vi "nipkg-updateControlFilePackageName.vi"(8 "error in (no error)":errorcluster, 9 "New Package Display Name":string, 10 "New Package Name":string, 11 "Package data":T1) -> (0 "error out":errorcluster, 3 "Package data out":T1)   [LabVIEW 2014, in "nipkg-build-system.lvlib"]
uses:
  nipkg-build-system.lvlib
  types/Package data.ctl
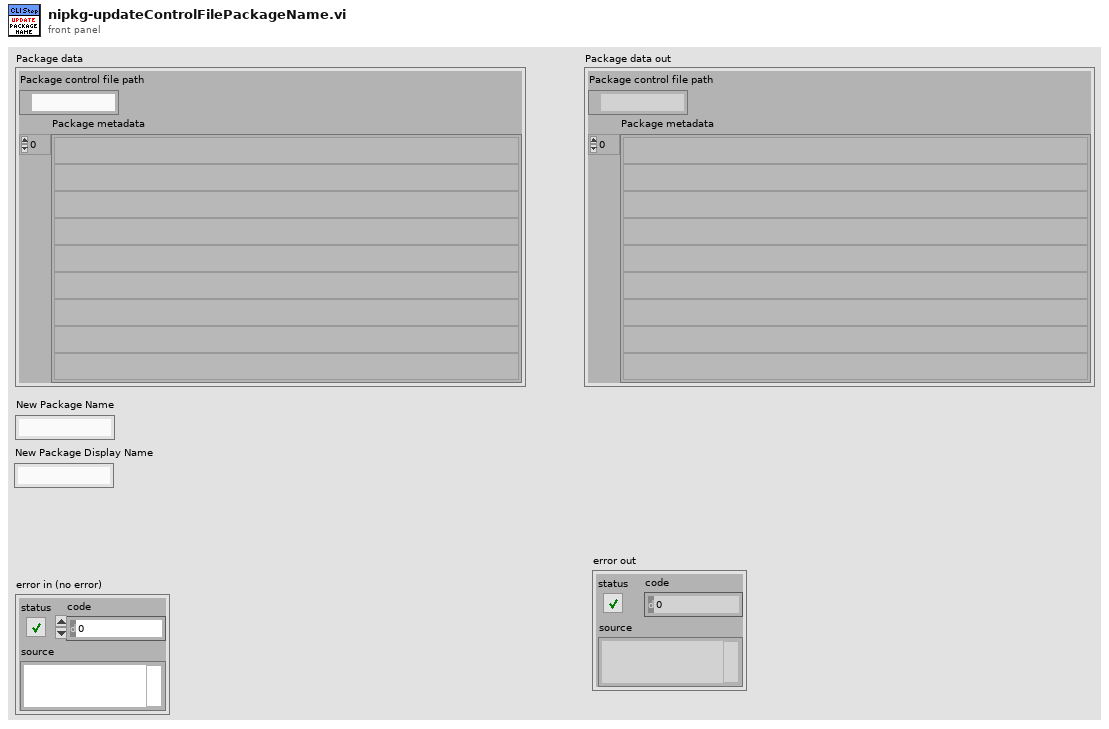
[diagram p1: front panel]
types:
  T1 = typedef "nipkg-build-system.lvlib/Package data.ctl" = cluster{"Package control file path":path, "Package metadata":string[]}
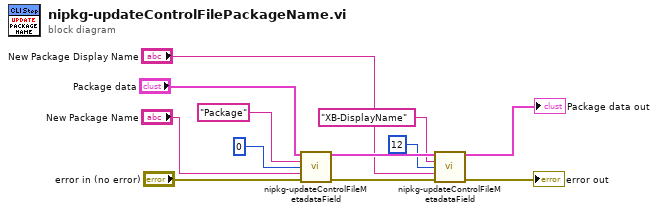
[diagram p0: block diagram]
diagram:
  n1 = call "nipkg-updateControlFileMetadataField.vi"("Package data"="Package data", "Metadata field name"="Package", "Metadata field index"=u8 0, "Metadata field value"="New Package Name", "error in (no error)"="error in (no error)") -> ("Package data out"=w6:T1, "error out"=w7:errorcluster)  [unwired: 9 in]
  n2 = call "nipkg-updateControlFileMetadataField.vi"("Package data"=w6, "Metadata field name"="XB-DisplayName", "Metadata field index"=u8 12, "Metadata field value"="New Package Display Name", "error in (no error)"=w7) -> ("Package data out"=→"Package data out":T1, "error out"=→"error out":errorcluster)  [unwired: 9 in]
